vi "FrequencyCalc.vi"(4 "Checkbox":bool, 6 "Number of teeth in gear":dbl, 7 "Period\n(s) in":dbl, 9 "dt":dbl, 10 "queue in":refnum<queue>, 11 "Queue in":refnum<queue>) -> (0 "Omega [RPM]":dbl(knob) scale=0.0..2000.0, 2 "Period\n(s) out":dbl, 3 "Signal Frequency (Hz)":dbl format="%#_13g", 5 "RPM 2":dbl)   [LabVIEW 2020]
panel:
  out "Numeric":dbl
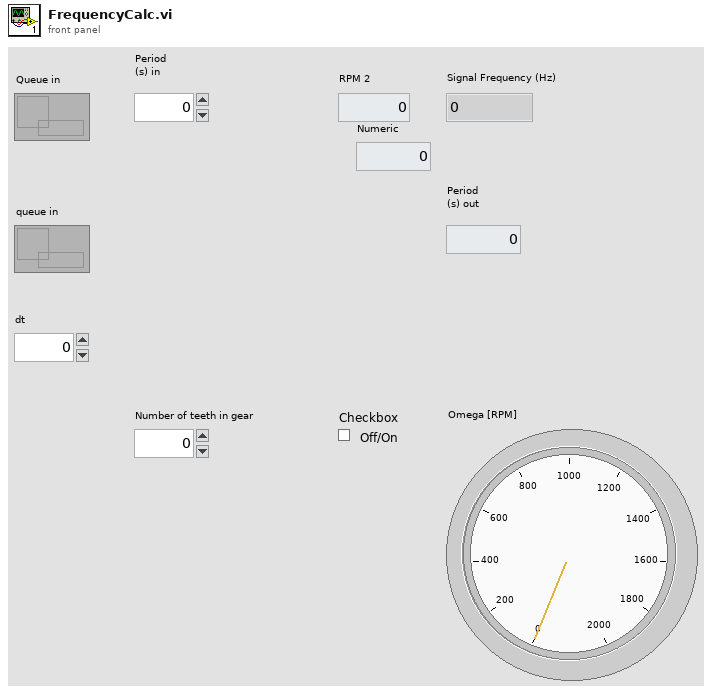
[diagram p1: front panel]
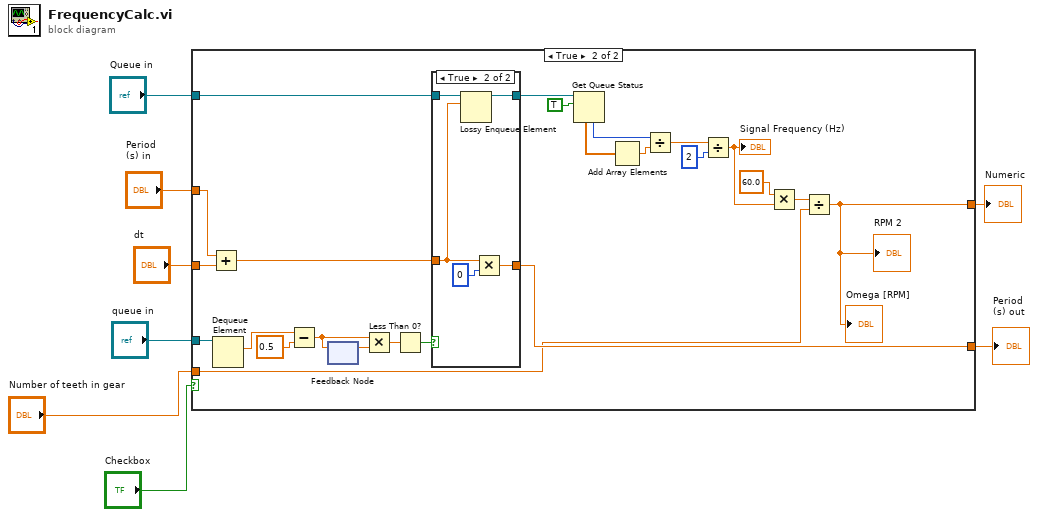
[diagram p0: block diagram]
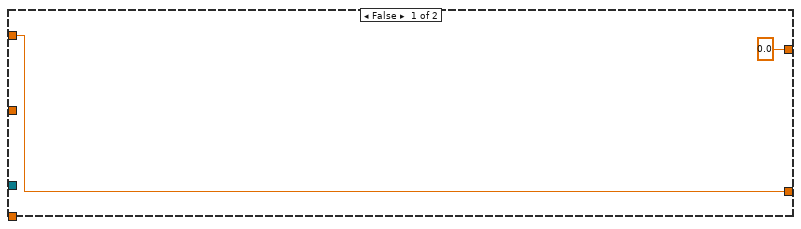
[diagram p2: hidden frame]
diagram:
  n1 = case shown="True" "Checkbox" {
    tunnel: "queue in" -> [_ w34]
    tunnel: "Queue in" -> [_ w28]
    tunnel: "Period\n(s) in" -> [w10 w18]
    tunnel: "dt" -> [_ w17]
    tunnel: [w10 w20] -> w6
    tunnel: "Number of teeth in gear" -> [_ w12]
    tunnel: [0.0 w11] -> w1
    frame False {
    }
    frame True {
      n2 = Add(x=w18, y=w17) -> (x+y=w16:dbl)
      n3 = Dequeue Element(queue=w34) -> (element=w33:dbl)  [unwired: 2 in, 3 out]
      n4 = Subtract(x=w33, y=0.5) -> (x-y=w31:dbl)
      n5 = feedback-in #1(w31) -> ()
      n6 = feedback #1() -> (w30:dbl)  [unwired: 1 in]
      n7 = Multiply(x=w31, y=w30) -> (x*y=w29:dbl)
      n8 = Less Than 0?(x=w29) -> (x < 0?=w19:bool)
      n9 = case shown="True" w19 {
        tunnel: w28 -> [w36 w40]
        tunnel: [w36 w39] -> w26
        tunnel: [w35 w38] -> w20
        tunnel: w16 -> [w35 w37]
        frame False {
        }
        frame True {
          n10 = Lossy Enqueue Element(queue=w40, element=w37) -> (queue out=w39:refnum<queue>)  [unwired: 1 in, 3 out]
          n11 = Multiply(x=w37, y=0) -> (x*y=w38:dbl)
        }
      }
      n12 = Get Queue Status(queue=w26, return elements? (F)=TRUE) -> (# elements in queue=w21:i32, elements=w25:dbl[])  [unwired: 1 in, 6 out]
      n13 = Add Array Elements(numeric array=w25) -> (sum=w22:dbl)
      n14 = Divide(x=w21, y=w22) -> (x/y=w23:dbl)
      n15 = Divide(x=w23, y=2) -> (x/y=w14:dbl)
      "Signal Frequency (Hz)" <- w14
      n16 = Multiply(x=60.0, y=w14) -> (x*y=w13:dbl)
      n17 = Divide(x=w13, y=w12) -> (x/y=w11:dbl)
      "RPM 2" <- w11
      "Omega [RPM]" <- w11
    }
  }
  "Period\n(s) out" <- w6
  "Numeric" <- w1
